vi "modbus slave全局.vi"() -> ()   [LabVIEW 2016]
panel:
  in  "执行结果反馈":u16[](array[numeric])
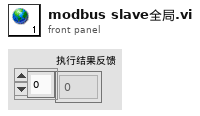
[diagram p1: front panel]
diagram:
